vi "NormalAttackerRoleCheckTacticChangeVSS.vi"(8 "error in (no error)":errorcluster, 9 "Game in":refnum<class "Game.lvclass">, 10 "Robot In":refnum<class "Robot.lvclass">, 11 "NormalAttackerRoleVSS in":refnum<class "NormalAttackerRoleVSS.lvclass">) -> (0 "error out":errorcluster, 2 "Tactic":T1(ring), 3 "NormalAttackerRoleVSS out":refnum<class "NormalAttackerRoleVSS.lvclass">)   [LabVIEW 2023, in "NormalAttackerRoleVSS.lvclass"]
uses:
  NormalAttackerRoleVSS.lvclass
  Robot_class/Robot.lvclass
  Game_class/Game.lvclass
  Game_class/Read BallRef.vi
  Ball_class/Ball.lvclass
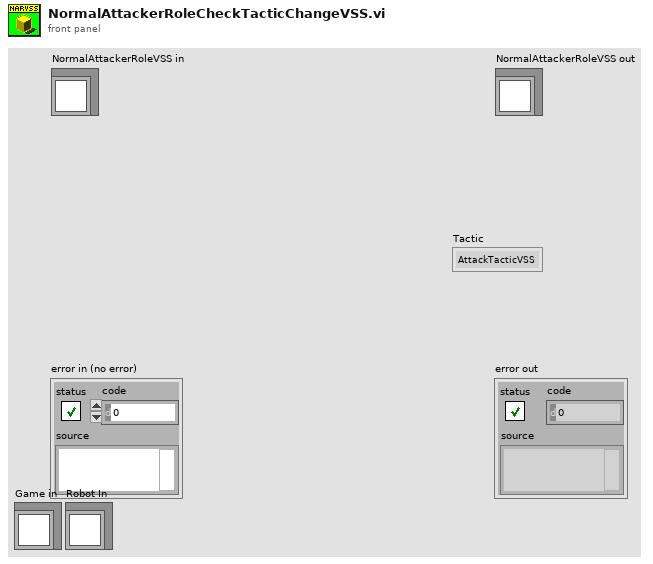
[diagram p1: front panel]
types:
  T1 = enum16{"AttackTacticVSS", "CounterAttackTacticVSS", "Exit"}
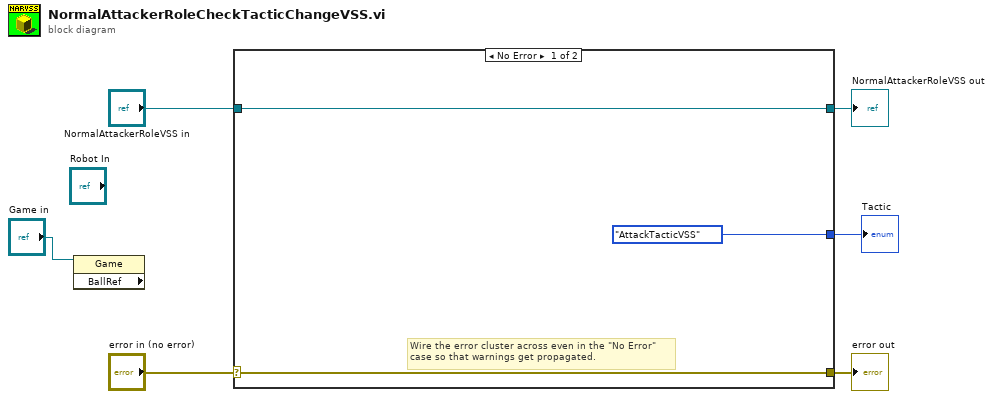
[diagram p0: block diagram]
diagram:
  n1 = property class="Game" props=["BallRef"](reference="Game in") -> ()  [unwired: 1 in, 3 out]
  n2 = case shown="No Error" "error in (no error)" {
    selector: "error in (no error)" -> [w8 w11]
    tunnel: [w8 w11] -> w5
    tunnel: [w9 w10] -> w3
    tunnel: "NormalAttackerRoleVSS in" -> [w9 w10]
    tunnel: [T1."AttackTacticVSS" ("Tactic") _] -> w1
    frame No Error {
      # "Wire the error cluster across even in the \"No Error\"\ncase so that warnings get propagated."
    }
    frame Error {
    }
  }
  "error out" <- w5
  "NormalAttackerRoleVSS out" <- w3
  "Tactic" <- w1
